vi "select_queue_path.vi"(7 "Control":enum16{"Invert", "Direct"}(ring), 8 "Message Queue 2":refnum<queue>, 11 "Message Queue":refnum<queue>) -> (0 "dup Message Queue 2":refnum<queue>, 3 "dup Message Queue":refnum<queue>)   [LabVIEW 2015]
uses:
  support/Message Queue/Message Cluster.ctl
  support/Message Queue/Message Queue.lvlib
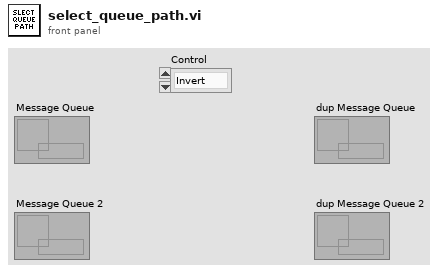
[diagram p1: front panel]
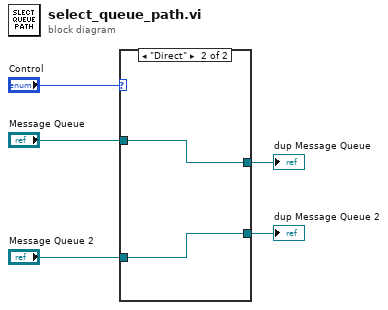
[diagram p0: block diagram]
diagram:
  n1 = case shown="\"Direct\"" "Control" {
    tunnel: "Message Queue" -> [w7 w9]
    tunnel: [w7 w8] -> w3
    tunnel: [w6 w9] -> w2
    tunnel: "Message Queue 2" -> [w6 w8]
    frame "Invert" {
    }
    frame "Direct" {
    }
  }
  "dup Message Queue" <- w2
  "dup Message Queue 2" <- w3
